vi "DisableCell.vi"(0 "MenuDisableCol in":refnum<class "MenuDisableCol.lvclass">, 1 "Col Array Ref in":refnum<vi>, 5 "Cell Position":T1, 7 "Table Data in":string[][](array[string]), 9 "Table CtlRef In":refnum<vi>, 11 "error in (no error)":errorcluster) -> (4 "MenuDisableCol out":refnum<class "MenuDisableCol.lvclass">, 8 "Table Data out":string[][](array[string]), 10 "Table CtlRef Out":refnum<vi>, 15 "error out":errorcluster)   [LabVIEW 2013, in "MenuDisableCol.lvclass"]
uses:
  MenuDisableCol.lvclass
  <vilib>/Utility/miscctls.llb/LVRowAndColumnTypeDef.ctl
  MenuCol/MenuCol.lvclass
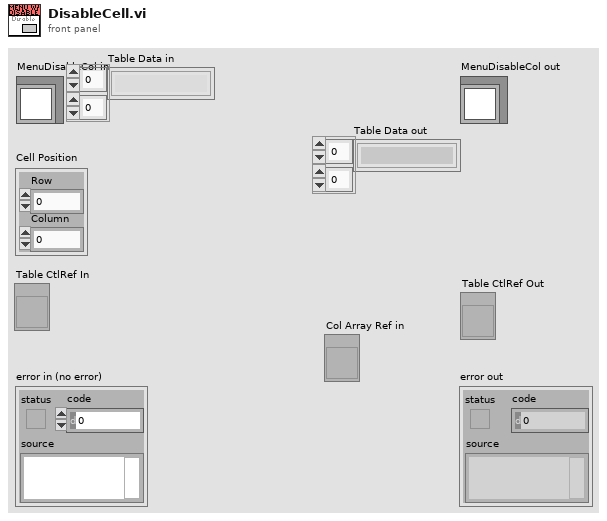
[diagram p1: front panel]
types:
  T1 = typedef "LVRowAndColumnTypeDef.ctl" = cluster{"Row":i32, "Column":i32}
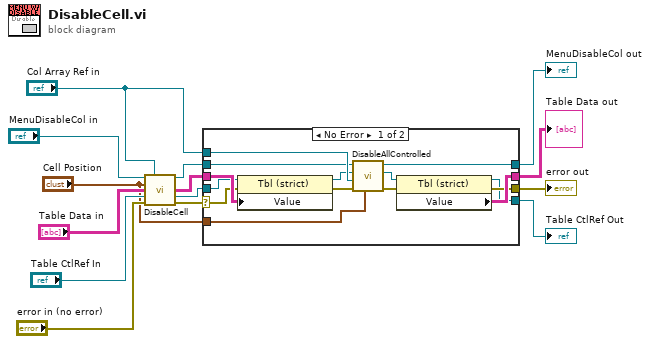
[diagram p0: block diagram]
diagram:
  n1 = call-parent "DisableCell.vi"("Column in"="MenuDisableCol in", "Col Array Ref in"="Col Array Ref in", "Cell Position"="Cell Position", "Table Data in"="Table Data in", "Table CtlRef In"="Table CtlRef In", "error in (no error)"="error in (no error)") -> ("Column out"=w7:refnum<class "MenuDisableCol.lvclass">, "Table Data out"=w1:string[][], "Table CtlRef Out"=w8:refnum<vi>, "error out"=w2:errorcluster)  [unwired: 6 in]
  n2 = case shown="No Error" w2 {
    selector: w2 -> [w17 w31]
    tunnel: "Cell Position" -> [w28 _]
    tunnel: "Col Array Ref in" -> [w27 _]
    tunnel: w8 -> [w18 w30]
    tunnel: w7 -> [w26 w29]
    tunnel: [w25 w32] -> w6
    tunnel: [w24 w31] -> w5
    tunnel: [w21 w30] -> w4
    tunnel: [w20 w29] -> w3
    tunnel: w1 -> [w19 w32]
    frame No Error {
      n3 = property class="Tbl (strict)"(reference=w18, error in=w17, "Value"=w19) -> (reference out=w15:refnum<vi>, error out=w16:errorcluster)
      n4 = call-dynamic "DisableAllControlled.vi"("Cell Position"=w28, "error in (no error)"=w16, "Col Array Ref in"=w27, "Table CtlRef in"=w15, "MenuDisableCol in"=w26) -> ("error out"=w23:errorcluster, "Table CtlRef out"=w22:refnum<vi>, "MenuDisableCol out"=w20:refnum<class "MenuDisableCol.lvclass">)  [unwired: 3 in, 1 out]
      n5 = property class="Tbl (strict)"(reference=w22, error in=w23) -> (reference out=w21:refnum<vi>, error out=w24:errorcluster, "Value"=w25:string[][])
    }
    frame Error {
    }
  }
  "error out" <- w5
  "Table CtlRef Out" <- w4
  "Table Data out" <- w6
  "MenuDisableCol out" <- w3
